vi "String to U8.vi"(11 "String":string) -> (3 "Numeric":u8)   [LabVIEW 2016, in "SLL String.lvlib"]
uses:
  SLL String.lvlib
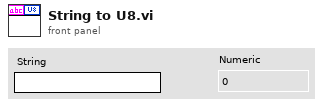
[diagram p1: front panel]
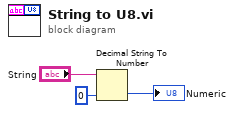
[diagram p0: block diagram]
diagram:
  n1 = Decimal String To Number(string="String", default (0L)=u8 0 ("default (0 I32)")) -> (number=→"Numeric":u8)  [unwired: 1 in, 1 out]
